vi "ATM_GetMessage.vi"(0 "Message Type":string, 1 "First Name":string, 2 "Last Name":string, 3 "Balance":dbl, 4 "User Input":dbl) -> (5 "ATM Message":string)   [LabVIEW 2020]
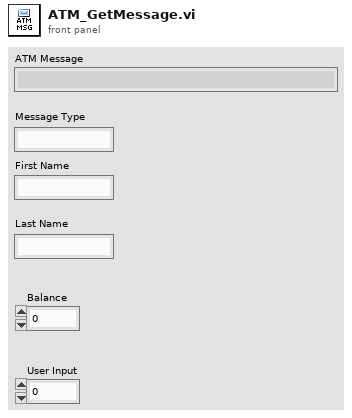
[diagram p1: front panel]
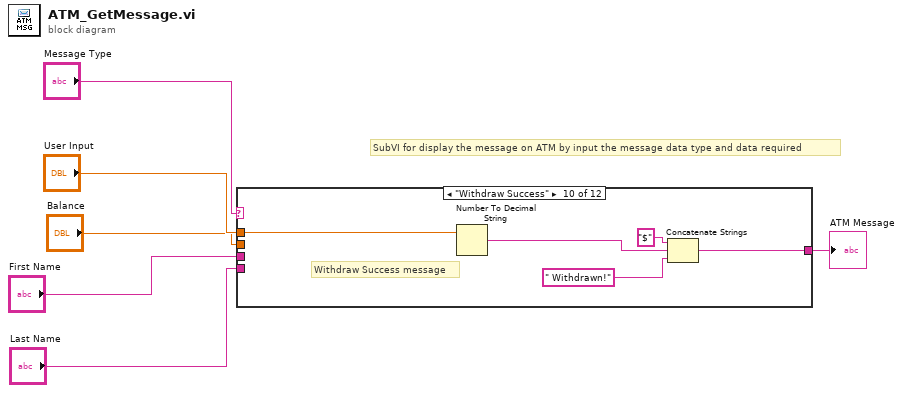
[diagram p0: block diagram]
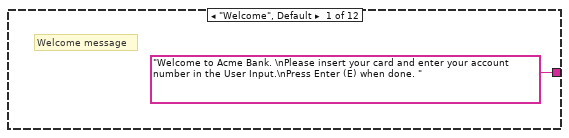
[diagram p2: hidden frame]
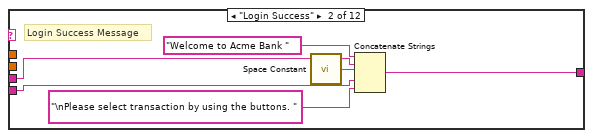
[diagram p3: hidden frame]
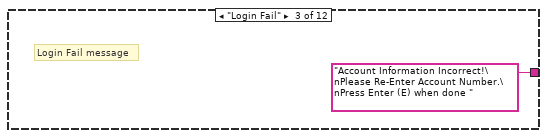
[diagram p4: hidden frame]
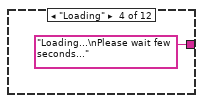
[diagram p5: hidden frame]
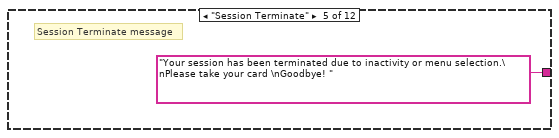
[diagram p6: hidden frame]
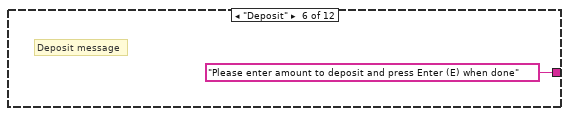
[diagram p7: hidden frame]
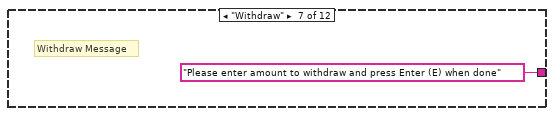
[diagram p8: hidden frame]
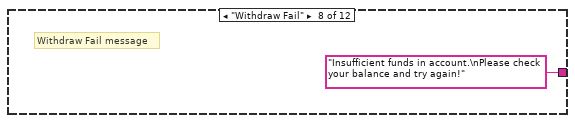
[diagram p9: hidden frame]
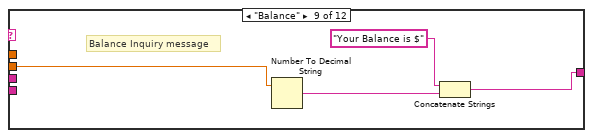
[diagram p10: hidden frame]
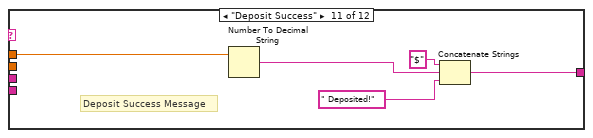
[diagram p11: hidden frame]
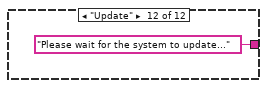
[diagram p12: hidden frame]
diagram:
  # "SubVI for display the message on ATM by input the message data type and data required"
  n1 = case shown="\"Withdraw Success\"" "Message Type" {
    tunnel: ["Welcome to Acme Bank. \nPlease insert your card and enter your account number in the User Input.\nPress Enter (E) when done. " ("ATM Message") w9 "Account Information Incorrect!\nPlease Re-Enter Account Number.\nPress Enter (E) when done " ("ATM Message") "Loading...\nPlease wait few seconds..." ("ATM Message") "Your session has been terminated due to inactivity or menu selection.\nPlease take your card \nGoodbye! " ("ATM Message") "Please enter amount to deposit and press Enter (E) when done" ("ATM Message") "Please enter amount to withdraw and press Enter (E) when done" ("ATM Message") "Insufficient funds in account.\nPlease check your balance and try again!" ("ATM Message") w23 w24 w29 "Please wait for the system to update..." ("ATM Message")] -> w6
    tunnel: "First Name" -> [_ w12 _ _ _ _ _ _ _ _ _ _]
    tunnel: "Last Name" -> [_ w11 _ _ _ _ _ _ _ _ _ _]
    tunnel: "User Input" -> [_ _ _ _ _ _ _ _ _ w28 w32 _]
    tunnel: "Balance" -> [_ _ _ _ _ _ _ _ w22 _ _ _]
    frame "Welcome", Default {
      # "Welcome message"
    }
    frame "Login Success" {
      # "Login Success Message"
      n2 = call <vilib>:"Space Constant.vi"() -> ("String"=w8:string)
      n3 = Concatenate Strings "Concatenate Strings"("Welcome to Acme Bank " ("string"), w12, w8, w11, "\nPlease select transaction by using the buttons. " ("string")) -> (w9:string)
    }
    frame "Login Fail" {
      # "Login Fail message"
    }
    frame "Loading" {
    }
    frame "Session Terminate" {
      # "Session Terminate message"
    }
    frame "Deposit" {
      # "Deposit message"
    }
    frame "Withdraw" {
      # "Withdraw Message"
    }
    frame "Withdraw Fail" {
      # "Withdraw Fail message"
    }
    frame "Balance" {
      # "Balance Inquiry message"
      n4 = Number To Decimal String(number=w22) -> (decimal integer string=w21:string)  [unwired: 1 in]
      n5 = Concatenate Strings "Concatenate Strings"("Your Balance is $" ("string"), w21) -> (w23:string)
    }
    frame "Withdraw Success" {
      # "Withdraw Success message"
      n6 = Number To Decimal String(number=w28) -> (decimal integer string=w27:string)  [unwired: 1 in]
      n7 = Concatenate Strings "Concatenate Strings"("$" ("string"), w27, " Withdrawn!" ("string")) -> (w24:string)
    }
    frame "Deposit Success" {
      # "Deposit Success Message"
      n8 = Number To Decimal String(number=w32) -> (decimal integer string=w31:string)  [unwired: 1 in]
      n9 = Concatenate Strings "Concatenate Strings"("$" ("string"), w31, " Deposited!" ("string")) -> (w29:string)
    }
    frame "Update" {
    }
  }
  "ATM Message" <- w6
